vi "Read Bias Voltages (V).vi"(11 "LCR-Measurement in":refnum<class "OTP_LCR_Meas.lvclass">) -> (2 "Bias Voltages (V)":dbl[](array[numeric]), 3 "LCR-Measurement out":refnum<class "OTP_LCR_Meas.lvclass">)   [LabVIEW 2020, in "OTP_LCR_Meas.lvclass"]
uses:
  OTP_LCR_Meas.lvclass
  OTP_LCR_Meas.lvclass/OTP_LCR_Meas.ctl
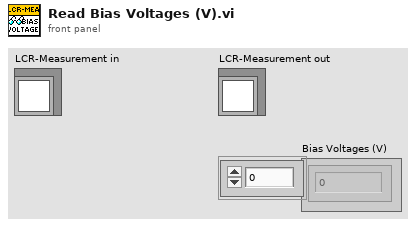
[diagram p1: front panel]
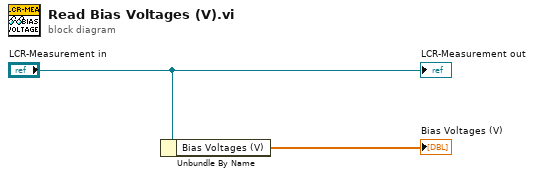
[diagram p0: block diagram]
diagram:
  n1 = Unbundle By Name("LCR-Measurement in") -> ("Bias Voltages (V)"=→"Bias Voltages (V)":dbl[])
  "LCR-Measurement out" <- "LCR-Measurement in"
